vi "Get_Auth_Code.vi"(8 "error in (no error)":errorcluster, 11 "OneNote in":refnum<class "OneNote.lvclass">) -> (0 "error out":errorcluster, 3 "OneNote out":refnum<class "OneNote.lvclass">)   [LabVIEW 2016, in "OneNote.lvclass"]
uses:
  OneNote.lvclass
  OneNote.lvclass/OneNote.ctl
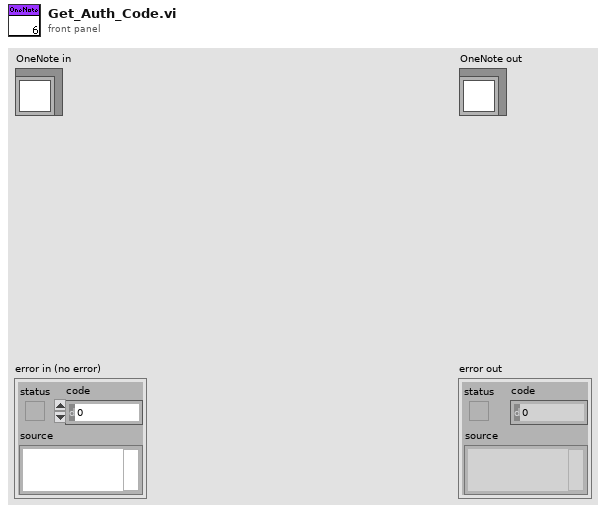
[diagram p1: front panel]
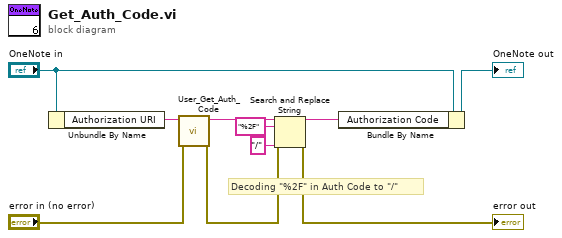
[diagram p0: block diagram]
diagram:
  # "Decoding \"%2F\" in Auth Code to \"/\""
  n1 = Unbundle By Name("OneNote in") -> ("Authorization URI"=w7:string)
  n2 = call "User_Get_Auth_Code.vi"("error in (no error)"="error in (no error)", "URL In"=w7) -> ("error out"=w2:errorcluster, "Auth Code"=w4:string)  [unwired: 8 in]
  n3 = Search and Replace String(input string=w4, search string="%2F", replace string="/" ("replace string (\"\")"), error in=w2) -> (result string=w3:string, error out=→"error out":errorcluster)  [unwired: 4 in, 2 out]
  n4 = Bundle By Name(cluster="OneNote in", "Authorization Code"=w3) -> (→"OneNote out":refnum<class "OneNote.lvclass">)
